vi "Read Stderr.vi"(5 "Username":string, 6 "Password":string, 7 "Address":string, 8 "Error In":errorcluster) -> (0 "Error Out":errorcluster)   [LabVIEW 2018, in "Tests.lvlib" / "Channel.lvlib"]
uses:
  Channel.lvlib
  <vilib>/addons/_JKI Toolkits/Caraya/classes/Test/Test.lvclass
  <vilib>/addons/_JKI Toolkits/Caraya/classes/Assert/Assert.lvclass
  src/Toolkit/Channel/Channel.lvclass
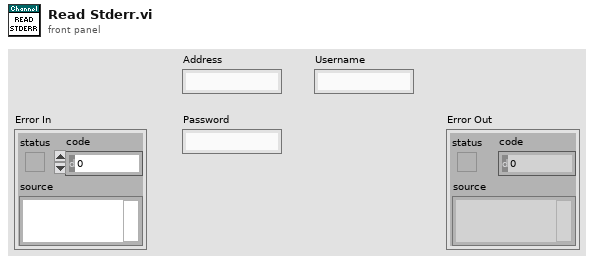
[diagram p1: front panel]
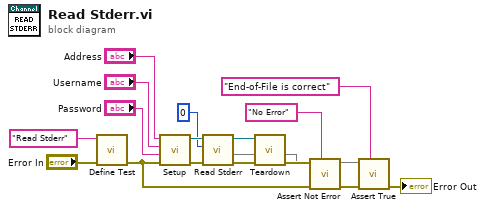
[diagram p0: block diagram]
diagram:
  n1 = call <vilib>:"Define Test.vi"("error in (no error)"="Error In", "Label (VI Title)"="Read Stderr") -> ("error out"=w13:errorcluster)  [unwired: 9 in]
  n2 = call "Setup.vi"("Error In"=w13, "Password"="Password", "Username"="Username", "Address"="Address") -> ("Error Out"=w8:errorcluster, "Channel"=w6:refnum<class "Channel.lvclass">)  [unwired: 6 in]
  n3 = call "Read Stderr.vi"("Error In"=w8, "Max Data Length"=0, "Channel In"=w6) -> ("Error Out"=w7:errorcluster, 1:w2, "Channel Out"=w5:refnum<class "Channel.lvclass">)  [unwired: 5 in, 1 out]
  n4 = call "Teardown.vi"("Error In"=w7, "Channel"=w5) -> ("Error Out"=w9:errorcluster)  [unwired: 9 in]
  n5 = call <vilib>:"Assert Not Error.vi"("Label"="No Error", "error in (no error)"=w13, "Not Error?"=w9) -> ("error out"=w14:errorcluster)  [unwired: 8 in]
  n6 = call <vilib>:"Assert True.vi"("Label"="End-of-File is correct", "error in (no error)"=w14, "True?"=w2) -> ("error out"=→"Error Out":errorcluster)  [unwired: 8 in]
